vi "1D Fit Rescale Fit Results (Stats).vi"(9 "Weighted":T1, 10 "Normalization Factor":dbl, 11 "Fit Results (Stats) in":T2[](array[typedef])) -> (3 "Fit Results (Stats) out":T2[](array[typedef]))   [LabVIEW 2021, in "Fits.lvlib"]
uses:
  Fits.lvlib
  Fit Results (statistics).ctl
  Non-linear Fitting Method v2.ctl
  Non-linear Fitting Algorithm.ctl
  IRF(X)PSED/Fit Weights Type v2.ctl
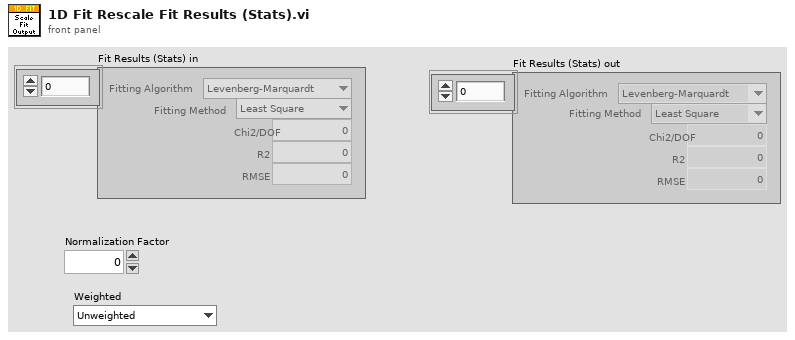
[diagram p1: front panel]
types:
  T1 = typedef "Fits.lvlib/Fit Weights Type v2.ctl" = enum16{"Unweighted", "1/Variance (Neyman)", "1/Variance (Pearson)", "Best of All"}
  T2 = typedef "Fits.lvlib/Fit Results (statistics).ctl" = cluster{"Chi2/DOF":dbl, "R2":dbl, "RMSE":dbl, "Fitting Method":T3, "Fitting Algorithm":T4}
  T3 = typedef "Fits.lvlib/Non-linear Fitting Method v2.ctl" = enum16{"Least Square", "Least Absolute Residual", "Bisquare", "MLE", "-", "Best of All"}
  T4 = typedef "Fits.lvlib/Non-linear Fitting Algorithm.ctl" = enum16{"Levenberg-Marquardt", "Trust-Region Dogleg"}
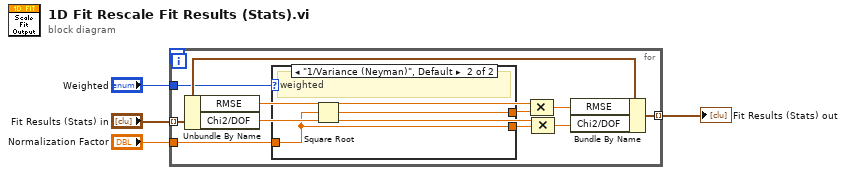
[diagram p0: block diagram]
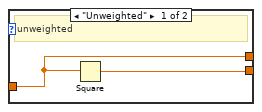
[diagram p2: hidden frame]
diagram:
  n1 = for {
    tunnel: "Fit Results (Stats) in" -> [w13] mode=indexing
    tunnel: "Normalization Factor" -> [w14]
    tunnel: [w6] -> w3 mode=indexing
    tunnel: "Weighted" -> [w5]
    n2 = Unbundle By Name(w13) -> ("RMSE"=w12:dbl, "Chi2/DOF"=w9:dbl)
    n3 = case shown="\"1/Variance (Neyman)\", Default" w5 {
      tunnel: w14 -> [w15 w17]
      tunnel: [w15 w18] -> w11
      tunnel: [w16 w17] -> w8
      frame "Unweighted" {
        # "unweighted"
        n4 = Square(x=w15) -> (x^2=w16:dbl)
      }
      frame "1/Variance (Neyman)", Default {
        # "weighted"
        n5 = Square Root(x=w17) -> (sqrt(x)=w18:dbl)
      }
    }
    n6 = Compound Arithmetic op=MULTIPLY(w12, w11) -> (w10:dbl)
    n7 = Compound Arithmetic op=MULTIPLY(w9, w8) -> (w7:dbl)
    n8 = Bundle By Name(cluster=w13, "RMSE"=w10, "Chi2/DOF"=w7) -> (w6:T2)
  }
  "Fit Results (Stats) out" <- w3
